vi "Read Waveform (Single) With Data Output.vi"(8 "error in (no error)":errorcluster, 9 "Timeout (10000 ms)":u32=10000, 10 "Source (1: Channel 1)":u16(ring)=1 items=["Channel 1"=1, "Channel 2"=2, "Channel 3"=3, "Channel 4"=4], 11 "VISA resource name":refnum<visa-resource-name>) -> (0 "error out":errorcluster, 2 "Waveform Data":waveform(dbl)(graph))   [LabVIEW 2021]
doc: "Initiates an acquisition on all channels that you enabled with the <B>Configure Channel</B> VI. The VI waits for the acquisition to complete and returns the waveform for the Source channel you specified. If the oscilloscope did not complete the acquisition within the time period you specify with the Timeout parameter, the VI returns a time out error. A common cause for a timeout error is the acquisition was not triggered. For example, the trigger level is out of range of the waveform.\n\nCall the <B>Fetch Waveform</B> VI to obtain the waveforms for each of the remaining enabled Source channels without initiating another acquisition.\n\nNote: If your instrument does not support auto compensation for probe attenuation, you may need to adjust the scaling of the Waveform Data accordingly. This is handled automatically in the <B>Configure Channel</B> VI or can be done manually by multiplying the Waveform Data by the probe attenuation."
uses:
  <vilib>/Waveform/WDTFileIO.llb/Export Waveform To Spreadsheet File.vi
  <instrlib>/Siglent SDS 1000 2000 Series/Siglent SDS 1000 2000 Series.lvlib
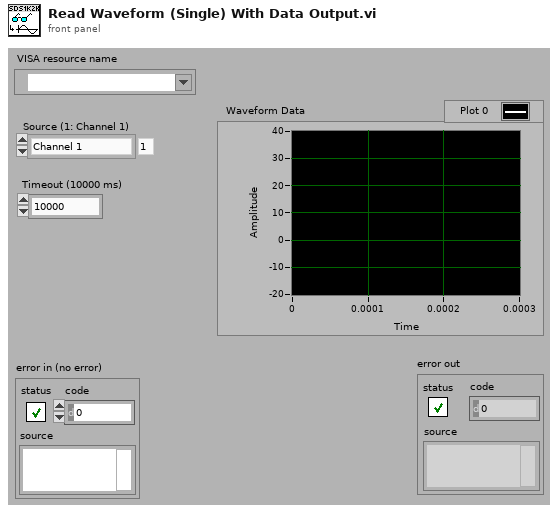
[diagram p1: front panel]
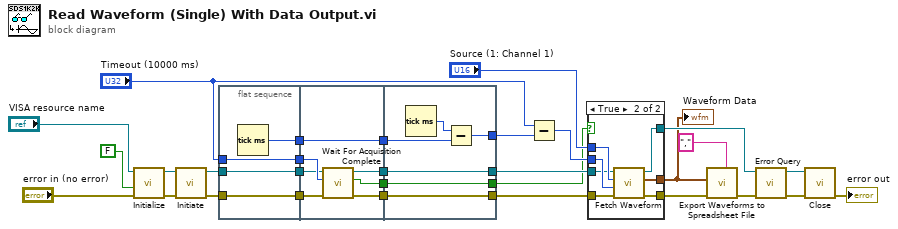
[diagram p0: block diagram]
diagram:
  n1 = call <instrlib>:"Initialize.vi"("error in (no error)"="error in (no error)", "Reset (True)"=FALSE, "VISA resource name"="VISA resource name") -> ("error out"=w7:errorcluster, "VISA resource name out"=w5:refnum<visa-resource-name>)  [unwired: 7 in]
  n2 = call <instrlib>:"Initiate.vi"("error in (no error)"=w7, "VISA resource name"=w5) -> ("error out"=w27:errorcluster, "VISA resource name out"=w28:refnum<visa-resource-name>)  [unwired: 8 in]
  n3 = flat-sequence {
    tunnel: "Timeout (10000 ms)" -> [w33]
    tunnel: [w33] -> w20
    tunnel: w28 -> [w32]
    tunnel: [w32] -> w19
    tunnel: w27 -> [w31]
    tunnel: [w31] -> w18
    tunnel: [w34] -> w17
    tunnel: w20 -> [w41]
    tunnel: w19 -> [w39]
    tunnel: w18 -> [w37]
    tunnel: [w36] -> w16
    tunnel: [w38] -> w15
    tunnel: [w40] -> w14
    tunnel: w17 -> [w35]
    tunnel: [w35] -> w13
    tunnel: [w44] -> w26
    tunnel: w16 -> [w44]
    tunnel: [w43] -> w22
    tunnel: w15 -> [w43]
    tunnel: [w45] -> w24
    tunnel: [w42] -> w21
    tunnel: w14 -> [w42]
    tunnel: w13 -> [w46]
    frame #0 {
      n4 = Tick Count (ms)() -> (millisecond timer value=w34:u32)
    }
    frame #1 {
      n5 = call <instrlib>:"Wait For Acquisition Complete.vi"("error in (no error)"=w37, "Timeout (10000 ms)"=w41, "VISA resource name"=w39) -> ("error out"=w36:errorcluster, "Complete"=w40:bool, "VISA resource name out"=w38:refnum<visa-resource-name>)  [unwired: 6 in]
    }
    frame #2 {
      n6 = Tick Count (ms)() -> (millisecond timer value=w47:u32)
      n7 = Subtract(x=w47, y=w46) -> (x-y=w45:u32)
    }
  }
  n8 = Subtract(x="Timeout (10000 ms)", y=w24) -> (x-y=w23:u32)
  n9 = case shown="True" w21 {
    tunnel: [_ w56] -> w10
    tunnel: [w49 w55] -> w30
    tunnel: [w48 w54] -> w11
    tunnel: "Source (1: Channel 1)" -> [_ w53]
    tunnel: w26 -> [w48 w52]
    tunnel: w23 -> [_ w51]
    tunnel: w22 -> [w49 w50]
    frame False {
    }
    frame True {
      n10 = call <instrlib>:"Fetch Waveform.vi"("error in (no error)"=w52, "Timeout (10000 ms)"=w51, "Source (1: Channel 1)"=w53, "VISA resource name"=w50) -> ("error out"=w54:errorcluster, "Waveform Graph"=w56:waveform(dbl), "VISA resource name out"=w55:refnum<visa-resource-name>)  [unwired: 5 in]
    }
  }
  "Waveform Data" <- w10
  n11 = call-poly <vilib>:"Export Waveforms to Spreadsheet File.vi"("delimiter (Tab)"=",", "error in (no error)"=w11, "waveform"=w10) -> ("error out"=w12:errorcluster)  [unwired: 7 in, 1 out]
  n12 = call <instrlib>:"Error Query.vi"("error in (no error)"=w12, "VISA resource name"=w30) -> ("error out"=w2:errorcluster, "VISA resource name out"=w3:refnum<visa-resource-name>)  [unwired: 6 in, 2 out]
  n13 = call <instrlib>:"Close.vi"("error in (no error)"=w2, "VISA resource name"=w3) -> ("error out"=→"error out":errorcluster)  [unwired: 9 in]
